vi "BuildSuiteTagName.vi"(9 "Suite Name":string, 10 "Parent Tag":string) -> (2 "Tag Name":string)   [LabVIEW 2017, in "ResultTree.lvclass"]
doc: "Returns the tag name for a test suite. If no parent tag is specified (\"\"), the tag name is the same as the suite name with prefix \"SUITE_\". If a parent tag is specified, however, the tag name is the same as the parent tag followed by a \"/\" and the name of the suite.\n\n<B>Examples</B>:\nparent: \"\"\nsuite: \"My suite\nresult: \"SUITE_My suite\"\n\nparent: \"SUITE_My suite\"\nsuite: \"Another suite\"\nresult: \"SUITE_My suite/Another suite\""
uses:
  ResultTree.lvclass
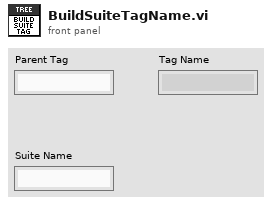
[diagram p1: front panel]
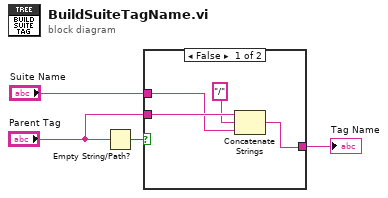
[diagram p0: block diagram]
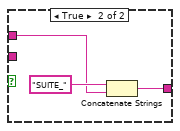
[diagram p2: hidden frame]
diagram:
  n1 = Empty String/Path?(string/path="Parent Tag") -> (empty?=w4:bool)
  n2 = case shown="False" w4 {
    tunnel: [w5 w10] -> w1
    tunnel: "Suite Name" -> [w6 w9]
    tunnel: "Parent Tag" -> [w8 _]
    frame False {
      n3 = Concatenate Strings(w8, "/" ("string"), w6) -> (w5:string)
    }
    frame True {
      n4 = Concatenate Strings("SUITE_", w9) -> (w10:string)
    }
  }
  "Tag Name" <- w1
